vi "DownloadDXF.vi"(8 "error in":errorcluster, 11 "Device In":T1) -> (0 "error out":errorcluster, 1 "DXF Text":string, 2 "Comm":T2, 3 "Device Out":T1)   [LabVIEW 2019]
uses:
  <userlib>/IoT Devices/_subVIs/HTTPComm.ctl
  <userlib>/Onshape/_SubVI/Cluster.ctl
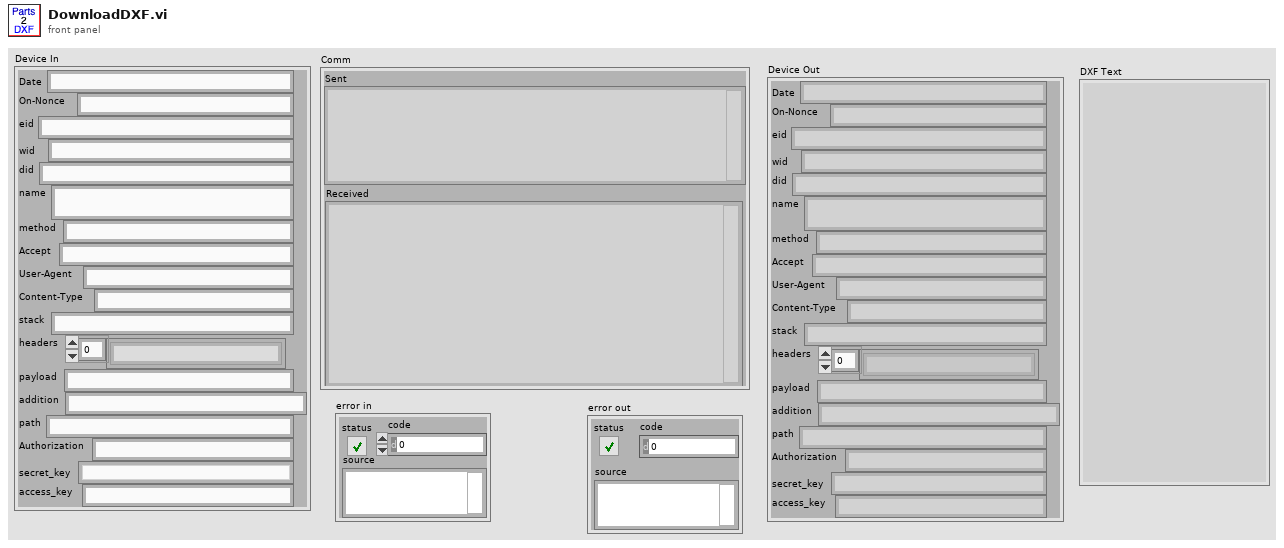
[diagram p1: front panel]
types:
  T1 = typedef "Cluster.ctl" = cluster{"Date":string, "On-Nonce":string, "eid":string, "wid":string, "did":string, "name":string, "method":string, "Accept":string, "User-Agent":string, "Content-Type":string, "stack":string, "headers":string[], "payload":string, "addition":string, "path":string, "Authorization":string, "secret_key":string, "access_key":string}
  T2 = typedef "HTTPComm.ctl" = cluster{"url":string, "sent headers":string, "sent body":string, "headers":string, "body":string, "Sent":string, "Received":string}
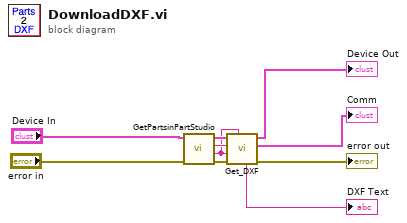
[diagram p0: block diagram]
diagram:
  n1 = call <userlib>:"GetPartsinPartStudio.vi"("error in"="error in", "Device In"="Device In") -> ("error out"=w5:errorcluster, "id"=w6:string, "documentMicroversion"=w7:string, "Device Out"=w8:T1)  [unwired: 6 in]
  n2 = call <userlib>:"Get_DXF.vi"("Save as"=w6, "error in"=w5, "Part Id"=w6, "microversion"=w7, "Device In"=w8) -> ("error out"=→"error out":errorcluster, "Comm"=→"Comm":T2, "Device Out"=→"Device Out":T1, "DXF Text"=→"DXF Text":string)  [unwired: 3 in]
